vi "SaveHands.vi"(8 "Error In":errorcluster, 11 ".NET Refnum in":refnum<k24>) -> (0 "Error Out":errorcluster, 3 "Hands":T1[](array[typedef]))   [LabVIEW 2014, in "LMH-Leap.lvlib"]
uses:
  LMH-Leap.lvlib
  Type Defs/Hand.ctl
  Type Defs/Vector.ctl
  Type Defs/Pointable.ctl
  Type Defs/Pointable Type.ctl
  Type Defs/Pointable Zone.ctl
  C:/github/makerhub/Leap/LabVIEW/vi.lib/LabVIEW Hacker/Leap/Private/Libs/LeapCSharp.NET3.5.dll
  LabVIEW Hacker/Leap/Private/Libs/LeapCSharp.NET3.5.dll
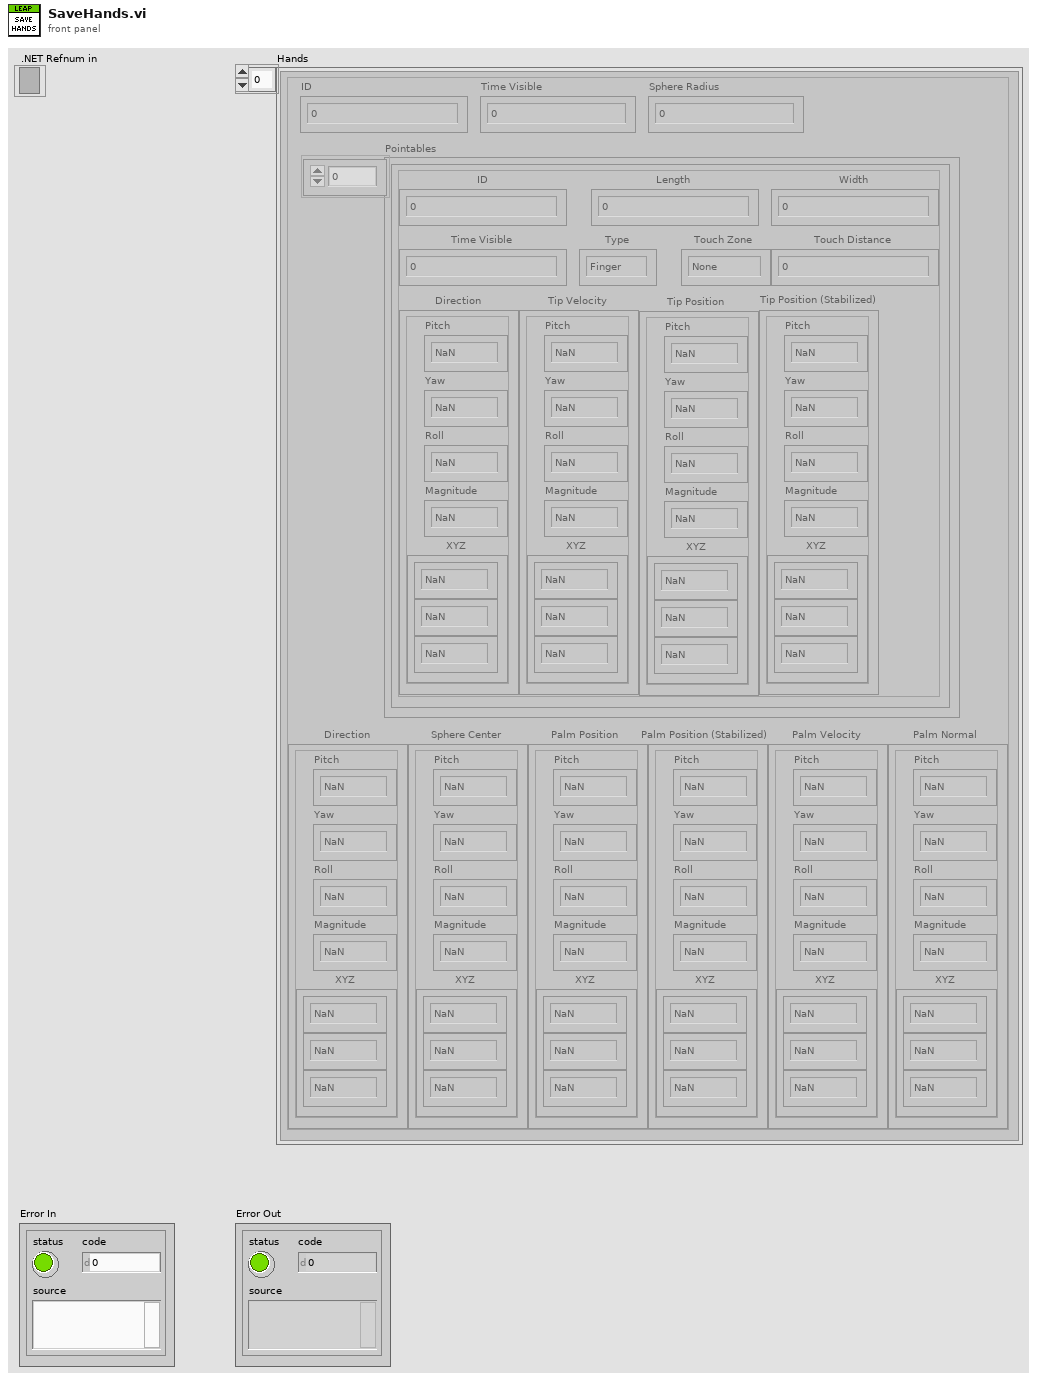
[diagram p1: front panel]
types:
  T1 = typedef "LMH-Leap.lvlib/Hand.ctl" = cluster{"Palm Normal":T2, "Palm Position":T2, "Palm Velocity":T2, "Direction":T2, "Palm Position (Stabilized)":T2, "Sphere Center":T2, "Pointables":T3[], "ID":i32, "Time Visible":sgl, "Sphere Radius":sgl}
  T2 = typedef "LMH-Leap.lvlib/Vector.ctl" = cluster{"Pitch":sgl, "Yaw":sgl, "Roll":sgl, "Magnitude":sgl, "XYZ":sgl[]}
  T3 = typedef "LMH-Leap.lvlib/Pointable.ctl" = cluster{"Type":T4, "Touch Zone":T5, "ID":i32, "Length":dbl, "Width":dbl, "Time Visible":dbl, "Touch Distance":dbl, "Direction":T2, "Tip Position":T2, "Tip Velocity":T2, "Tip Position (Stabilized)":T2}
  T4 = typedef "LMH-Leap.lvlib/Pointable Type.ctl" = enum16{"Finger", "Tool"}
  T5 = typedef "LMH-Leap.lvlib/Pointable Zone.ctl" = enum16{"None", "Hovering", "Touching"}
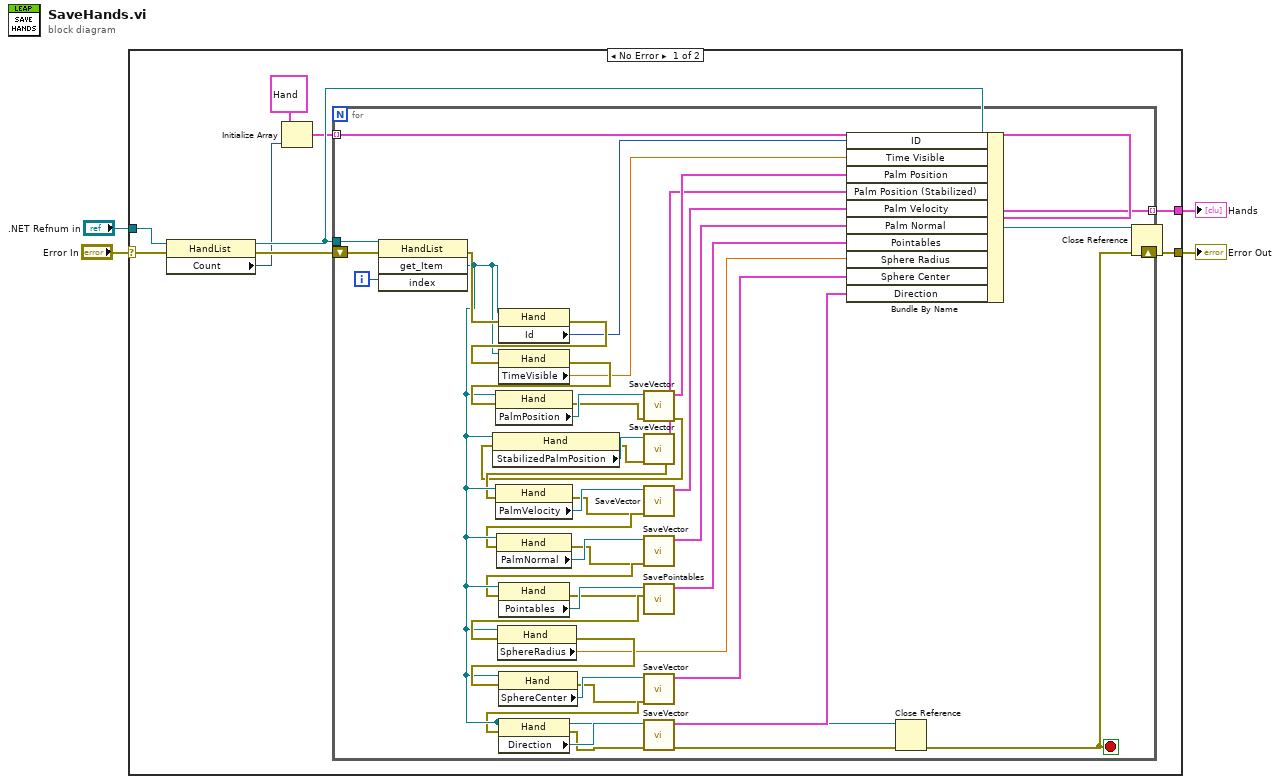
[diagram p0: block diagram]
diagram:
  n1 = case shown="No Error" "Error In" {
    selector: "Error In" -> [w7 w57]
    tunnel: [w12 _] -> w4
    tunnel: ".NET Refnum in" -> [w8 _]
    tunnel: [w5 w57] -> w2
    frame No Error {
      n2 = property class="HandList"(reference=w8, error in=w7) -> (reference out=w13:refnum<k24>, error out=w14:errorcluster, "Count"=w9:i32)
      n3 = Initialize Array(T1 {"Palm Normal"={"Pitch"=0.0, "Yaw"=0.0, "Roll"=0.0, "Magnitude"=0.0, "XYZ"=[]}, "Palm Position"={"Pitch"=0.0, "Yaw"=0.0, "Roll"=0.0, "Magnitude"=0.0, "XYZ"=[]}, "Palm Velocity"={"Pitch"=0.0, "Yaw"=0.0, "Roll"=0.0, "Magnitude"=0.0, "XYZ"=[]}, "Direction"={"Pitch"=0.0, "Yaw"=0.0, "Roll"=0.0, "Magnitude"=0.0, "XYZ"=[]}, "Palm Position (Stabilized)"={"Pitch"=0.0, "Yaw"=0.0, "Roll"=0.0, "Magnitude"=0.0, "XYZ"=[]}, "Sphere Center"={"Pitch"=0.0, "Yaw"=0.0, "Roll"=0.0, "Magnitude"=0.0, "XYZ"=[]}, "Pointables"=[], "ID"=0, "Time Visible"=0.0, "Sphere Radius"=0.0} ("Hand"), w9) -> (w11:T1[])
      n4 = for {
        tunnel: w13 -> [w49]
        tunnel: w11 -> [w47] mode=indexing
        tunnel: [w45] -> w12 mode=indexing
        shift-right: [w41] -> w6
        shift-left: w14 -> [w50]
        i -> [w48]
        stop <- w41 stop-if-true
        n5 = invoke class="HandList" method="get_Item"(reference=w49, error in=w50, "index"=w48) -> (error out=w54:errorcluster, "get_Item"=w28:refnum<k24>)  [unwired: 1 in, 2 out]
        n6 = property class="Hand"(reference=w28, error in=w54) -> (error out=w53:errorcluster, "Id"=w46:i32)  [unwired: 1 out]
        n7 = property class="Hand"(reference=w28, error in=w53) -> (error out=w51:errorcluster, "TimeVisible"=w40:sgl)  [unwired: 1 out]
        n8 = property class="Hand"(reference=w28, error in=w51) -> (error out=w16:errorcluster, "PalmPosition"=w39:refnum<k24>)  [unwired: 1 out]
        n9 = call "SaveVector.vi"("error in (no error)"=w16, "Leap Vector"=w39) -> ("error out"=w15:errorcluster, "Vector"=w37:T2)  [unwired: 8 in]
        n10 = property class="Hand"(reference=w28, error in=w15) -> (error out=w17:errorcluster, "StabilizedPalmPosition"=w38:refnum<k24>)  [unwired: 1 out]
        n11 = call "SaveVector.vi"("error in (no error)"=w17, "Leap Vector"=w38) -> ("error out"=w18:errorcluster, "Vector"=w36:T2)  [unwired: 8 in]
        n12 = property class="Hand"(reference=w28, error in=w18) -> (error out=w19:errorcluster, "PalmVelocity"=w44:refnum<k24>)  [unwired: 1 out]
        n13 = call "SaveVector.vi"("error in (no error)"=w19, "Leap Vector"=w44) -> ("error out"=w20:errorcluster, "Vector"=w35:T2)  [unwired: 8 in]
        n14 = property class="Hand"(reference=w28, error in=w20) -> (error out=w21:errorcluster, "PalmNormal"=w43:refnum<k24>)  [unwired: 1 out]
        n15 = call "SaveVector.vi"("error in (no error)"=w21, "Leap Vector"=w43) -> ("error out"=w22:errorcluster, "Vector"=w34:T2)  [unwired: 8 in]
        n16 = property class="Hand"(reference=w28, error in=w22) -> (error out=w32:errorcluster, "Pointables"=w33:refnum<k24>)  [unwired: 1 out]
        n17 = call "SavePointables.vi"("error in (no error)"=w32, "Leap Pointables"=w33) -> ("error out"=w52:errorcluster, "Pointables"=w23:T3[])  [unwired: 8 in]
        n18 = property class="Hand"(reference=w28, error in=w52) -> (error out=w55:errorcluster, "SphereRadius"=w31:sgl)  [unwired: 1 out]
        n19 = property class="Hand"(reference=w28, error in=w55) -> (error out=w24:errorcluster, "SphereCenter"=w42:refnum<k24>)  [unwired: 1 out]
        n20 = call "SaveVector.vi"("error in (no error)"=w24, "Leap Vector"=w42) -> ("error out"=w25:errorcluster, "Vector"=w30:T2)  [unwired: 8 in]
        n21 = property class="Hand"(reference=w28, error in=w25) -> (error out=w26:errorcluster, "Direction"=w29:refnum<k24>)  [unwired: 1 out]
        n22 = call "SaveVector.vi"("error in (no error)"=w26, "Leap Vector"=w29) -> ("error out"=w27:errorcluster, "Vector"=w56:T2)  [unwired: 8 in]
        n23 = Bundle By Name(cluster=w47, "ID"=w46, "Time Visible"=w40, "Palm Position"=w37, "Palm Position (Stabilized)"=w36, "Palm Velocity"=w35, "Palm Normal"=w34, "Pointables"=w23, "Sphere Radius"=w31, "Sphere Center"=w30, "Direction"=w56) -> (w45:T1)
        n24 = Close Reference(reference=w28, error in (no error)=w27) -> (error out=w41:errorcluster)
      }
      n25 = Close Reference(reference=w13, error in (no error)=w6) -> (error out=w5:errorcluster)
    }
    frame Error {
    }
  }
  "Hands" <- w4
  "Error Out" <- w2
